vi "input.vi"(8 "error in":errorcluster, 10 "input allocation":T1, 11 "module in":refnum<class "sample module runtime.lvclass">) -> (0 "error out":errorcluster, 2 "input data":T1, 3 "module out":refnum<class "sample module runtime.lvclass">)   [LabVIEW 2013, in "sample module runtime.lvclass"]
doc: "Provides an interface for reading data from a module at runtime. While this interface performs no operations, a child should provide an override which may read from any open sessions, references, or interfaces."
uses:
  sample module runtime.lvclass
  <vilib>/NI/Tag Bus/table/data table.ctl
  <vilib>/NI/Tag Bus/table/data table.lvlib
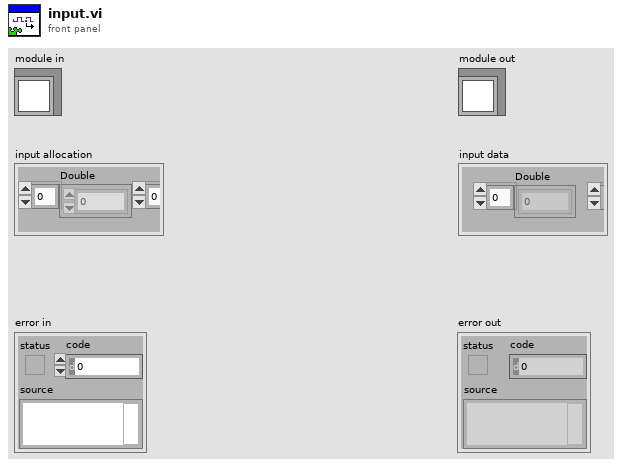
[diagram p1: front panel]
types:
  T1 = typedef "tag bus.lvlib/data table.lvlib/data table.ctl" = cluster{"Double":dbl[], "Single":sgl[], "I64":i64[], "I32":i32[], "I16":i16[], "I8":i8[], "U64":u64[], "U32":u32[], "U16":u16[], "U8":u8[], "Boolean":bool[], "String":string[], "Array of Double":cluster{"DBL Array":dbl[]}[], "Array of Single":cluster{"SGL Array":sgl[]}[], "Array of I64":cluster{"I64 Array":i64[]}[], "Array of I32":cluster{"I32 Array":i32[]}[], "Array of I16":cluster{"I16 Array":i16[]}[], "Array of I8":cluster{"I8 Array":i8[]}[], "Array of U64":cluster{"U64 Array":u64[]}[], "Array of U32":cluster{"U32 Array":u32[]}[], "Array of U16":cluster{"U16 Array":u16[]}[], "Array of U8":cluster{"U8 Array":u8[]}[], "Array of Boolean":cluster{"Boolean Array":bool[]}[], "Array of String":cluster{"String Array":string[]}[]}
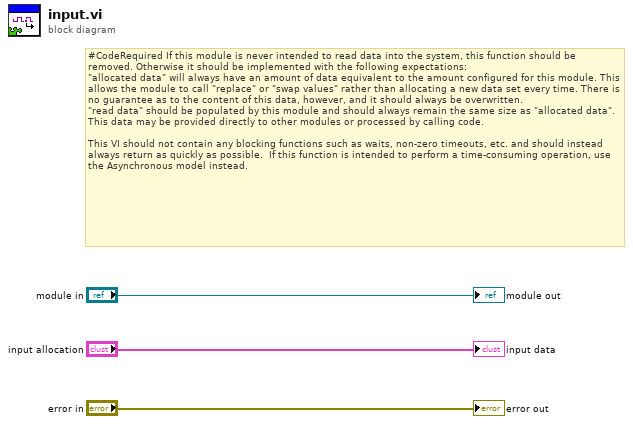
[diagram p0: block diagram]
diagram:
  # "#CodeRequired If this module is never intended to read data into the system, this function should be removed. Otherwise it should be implemented with the following expectations:\n\"allocated data\" will always have an amount of data equivalent to the amount configured for this module. This allows the module to call \"replace\" or \"swap values\" rather than allocating a new data set every time. There is no guarantee as to the content of this data, however, and it should always be overwritten.\n\"read data\" should be populated by this module and should always remain the same size as \"allocated data\". This data may be provided directly to other modules or processed by calling code.\n\nThis VI should not contain any blocking functions such as waits, non-zero timeouts, etc. and should instead always return as quickly as possible.  If this function is intended to perform a time-consuming operation, use the Asynchronous model instead."
  "error out" <- "error in"
  "module out" <- "module in"
  "input data" <- "input allocation"
